vi "SPI_SetChipSelectActiveState.vi"(5 "Device":i32, 6 "CS active state":bool, 7 "Bus":i32=1, 8 "error in":errorcluster) -> (0 "error out":errorcluster)   [LabVIEW 2014, in "GPIO.lvlib"]
doc: "Sets the active state of the Chip Select pin for the specified SPI device, default is active low."
uses:
  GPIO.lvlib
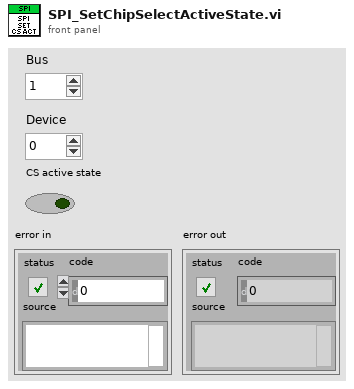
[diagram p1: front panel]
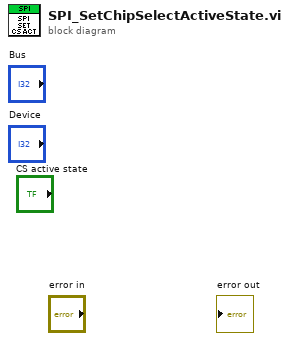
[diagram p0: block diagram]
diagram:
